vi "r_cent.vi"(1 "constraints cluster":T1, 2 "lmd_input":dbl[](array[numeric]), 3 "q_input":dbl[](array[numeric]), 4 "inv_t":dbl) -> (0 "central residual":dbl[](array[numeric]))   [LabVIEW 2019]
panel:
  # "input : constraints cluster\n            q_input\n            lmd_input\n            inv_t"
  # "output : central residual, \n               matrix, m*1"
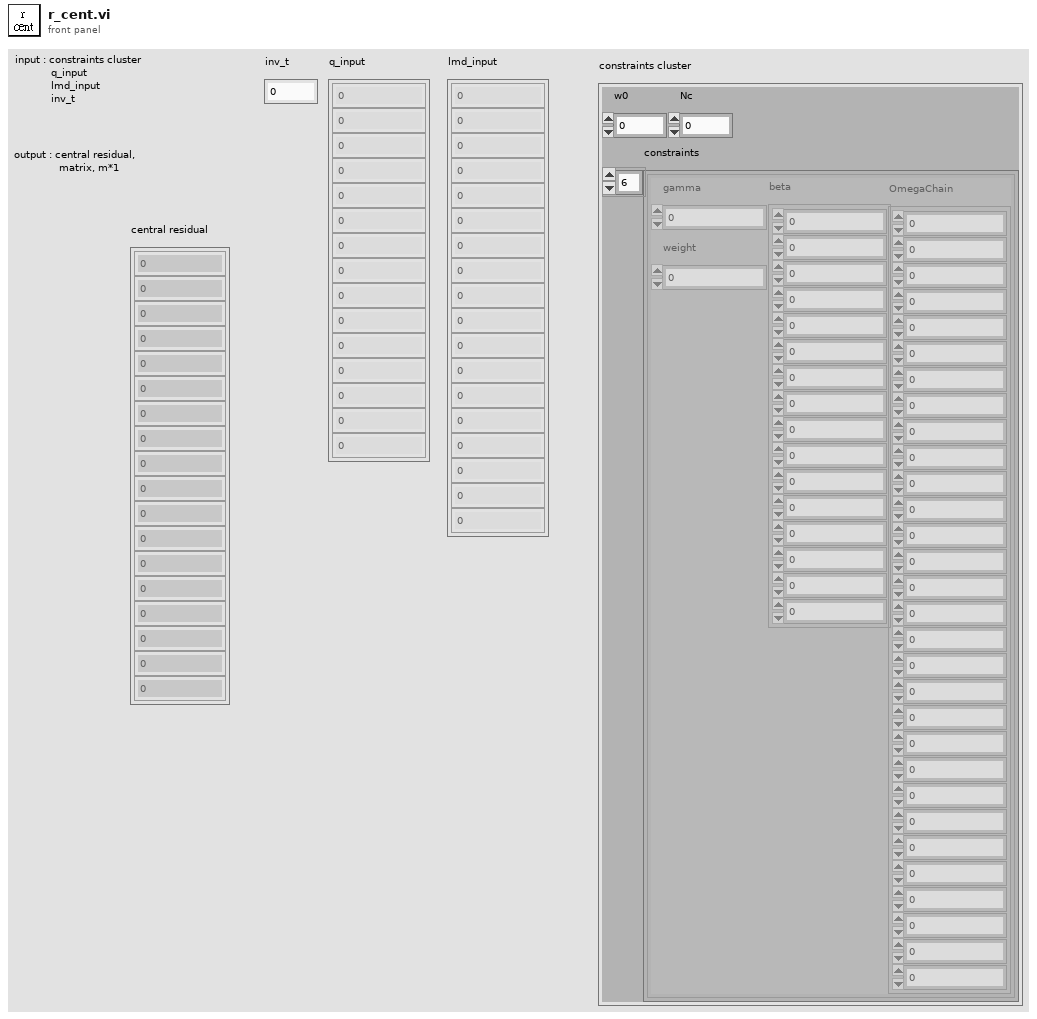
[diagram p1: front panel]
types:
  T1 = cluster{"w0":dbl, "constraints":cluster{"beta":dbl[], "gamma":dbl, "OmegaChain":dbl[], "weight":dbl}[], "Nc":i32}
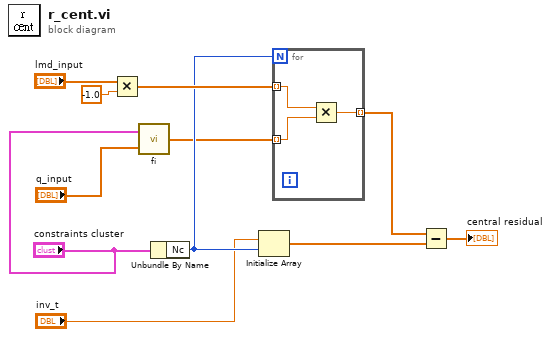
[diagram p0: block diagram]
diagram:
  n1 = Multiply(x="lmd_input", y=-1.0) -> (x*y=w9:dbl[])
  n2 = call "fi.vi"("q_input"="q_input", "constraints cluster"="constraints cluster") -> ("fi"=w5:dbl[])
  n3 = Unbundle By Name("constraints cluster") -> ("Nc"=w8:i32)
  n4 = Initialize Array("inv_t", w8) -> (w2:dbl[])
  n5 = for {
    N: w8 -> [_]
    tunnel: w9 -> [w14] mode=indexing
    tunnel: w5 -> [w13] mode=indexing
    tunnel: [w12] -> w4 mode=indexing
    n6 = Multiply(x=w14, y=w13) -> (x*y=w12:dbl)
  }
  n7 = Subtract(x=w4, y=w2) -> (x-y=→"central residual":dbl[])
